vi "删除启动项.vi"(8 "error in (no error)":errorcluster caption="错误输入（无错误）") -> (0 "error out":errorcluster caption="错误输出", 3 "删除标记":bool)   [LabVIEW 2016, in "Alarm interface.lvlib" / "wxpusher.lvlib"]
uses:
  wxpusher.lvlib
  <vilib>/registry/registry.llb/Registry RtKey.ctl
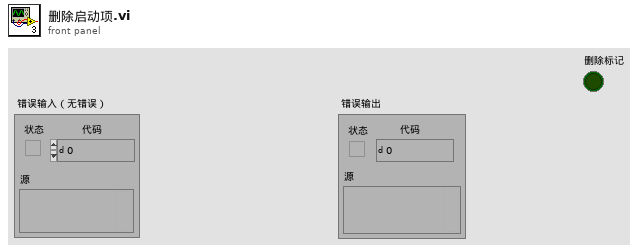
[diagram p1: front panel]
types:
  T1 = typedef "Registry RtKey.ctl" = enum32{"HKEY_CLASSES_ROOT", "HKEY_CURRENT_USER", "HKEY_LOCAL_MACHINE", "HKEY_USERS", "HKEY_PERFORMANCE_DATA", "HKEY_CURRENT_CONFIG", "HKEY_DYN_DATA"}
  T2 = typedef "Registry refnum.ctl" = refnum<k1>
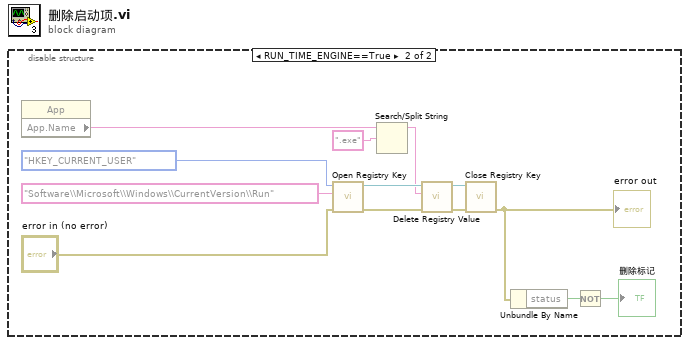
[diagram p0: block diagram]
diagram:
  n1 = disable-structure shown="RUN_TIME_ENGINE==True" {
    frame condition #0 (active) {
    }
    frame condition #1 {
      n2 = property class="App"() -> ("App.Name"=w2:string)  [unwired: 2 in, 2 out]
      n3 = call <vilib>:"Open Registry Key.vi"("error in (no error)"="error in (no error)", "subkey"="Software\\Microsoft\\Windows\\CurrentVersion\\Run", "root key (HKEY_LOCAL_MACHINE)"=Registry_RtKey."HKEY_CURRENT_USER") -> ("error out"=w8:errorcluster, "refnum out"=w10:T2)  [unwired: 7 in]
      n4 = Search/Split String(string=w2, search string/char (-)=".exe" ("搜索字符串/字符(-)")) -> (substring before match=w1:string)  [unwired: 1 in, 2 out]
      n5 = call <vilib>:"Delete Registry Value.vi"("error in (no error)"=w8, "value"=w1, "refnum"=w10) -> ("error out"=w7:errorcluster, "refnum out"=w9:T2)  [unwired: 7 in]
      n6 = call <vilib>:"Close Registry Key.vi"("error in (no error)"=w7, "refnum"=w9) -> ("error out"=w5:errorcluster)  [unwired: 5 in]
      "error out" <- w5
      n7 = Unbundle By Name(w5) -> ("status"=w4:bool)
      n8 = Not(x=w4) -> (.not. x?=→"删除标记":bool)
    }
  }
